vi "Exemple_Model_Selection_KFold.vi"() -> ()   [LabVIEW 2020]
panel:
  out "Split":T1(array[cluster])
  out "error out":errorcluster caption="sortie d'erreur"
  in  "KFold":T2={"n_splits"=2, "shuffle"=FALSE, "random_state"=-1} {"random_state" min=-1}
  in  "error in (no error)":errorcluster caption="entrée d'erreur (pas d'erreur)"
  in  "Groups":string[][](array[string])
  in  "y":string[][](array[string])=[["1"], ["2"], ["3"], ["4"]]
  in  "X":string[][](array[string])=[["1", "2"], ["3", "4"], ["1", "2"], ["3", "4"]]
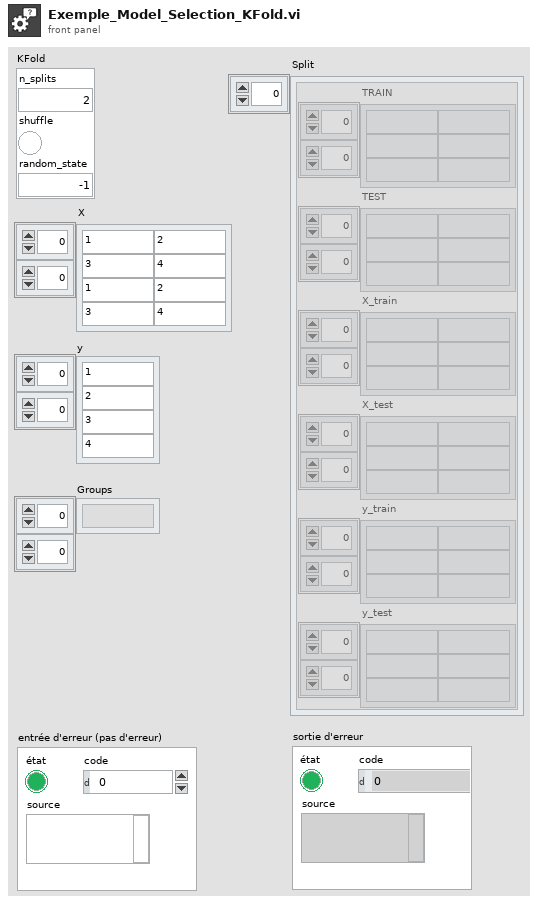
[diagram p1: front panel]
types:
  T1 = cluster{"TRAIN":string[][], "TEST":string[][], "X_train":string[][], "X_test":string[][], "y_train":string[][], "y_test":string[][]}[]
  T2 = cluster{"n_splits":i32, "shuffle":bool, "random_state":i32}
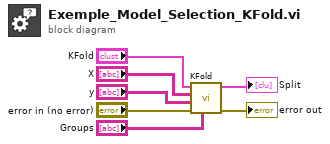
[diagram p0: block diagram]
diagram:
  n1 = call "KFold.vi"("Groups"="Groups", "error in (no error)"="error in (no error)", "y"="y", "X"="X", "KFold"="KFold") -> ("error out"=→"error out":errorcluster, "Split"=→"Split":T1)  [unwired: 5 in]
